vi "Coerce I64.vi"(4 "Rounding Mode (Round to Nearest))":T1, 8 "Value":i64, 9 "Increment":i64, 10 "Maximum":i64, 11 "Minimum":i64) -> (3 "Coerced Value":i64)   [LabVIEW 2020]
uses:
  Rounding Mode.ctl
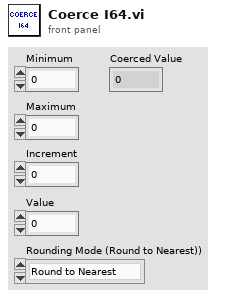
[diagram p1: front panel]
types:
  T1 = typedef "Rounding Mode.ctl" = enum16{"Round to Nearest", "Round to Lowest", "Round to Highest"}
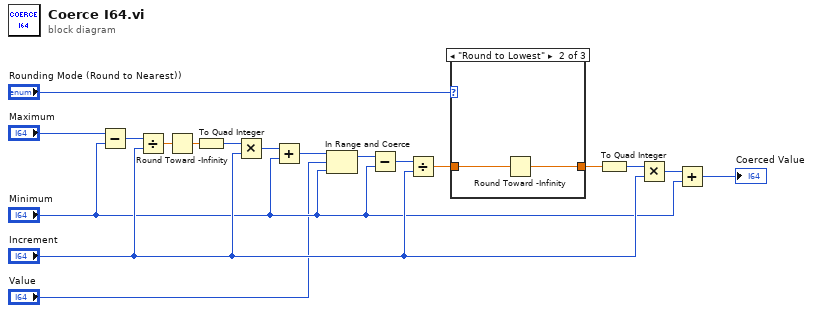
[diagram p0: block diagram]
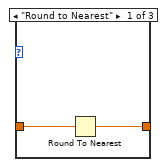
[diagram p2: hidden frame]
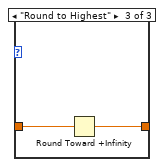
[diagram p3: hidden frame]
diagram:
  n1 = Subtract(x="Maximum", y="Minimum") -> (x-y=w14:i64)
  n2 = Divide(x=w14, y="Increment") -> (x/y=w13:dbl)
  n3 = Round Toward -Infinity(1:w13) -> (0:w8:dbl)
  n4 = To Quad Integer(1:w8) -> (0:w7:i64)
  n5 = Multiply(x=w7, y="Increment") -> (x*y=w6:i64)
  n6 = Add(x=w6, y="Minimum") -> (x+y=w10:i64)
  n7 = In Range and Coerce(upper limit=w10, x="Value", lower limit="Minimum") -> (coerced(x)=w16:i64)  [unwired: 1 out]
  n8 = Subtract(x=w16, y="Minimum") -> (x-y=w17:i64)
  n9 = Divide(x=w17, y="Increment") -> (x/y=w18:dbl)
  n10 = case shown="\"Round to Lowest\"" "Rounding Mode (Round to Nearest))" {
    tunnel: w18 -> [w20 w22 w24]
    tunnel: [w19 w21 w23] -> w4
    frame "Round to Nearest" {
      n11 = Round To Nearest(number=w20) -> (nearest integer value=w19:dbl)
    }
    frame "Round to Lowest" {
      n12 = Round Toward -Infinity(1:w22) -> (0:w21:dbl)
    }
    frame "Round to Highest" {
      n13 = Round Toward +Infinity(x=w24) -> (ceil(x): smallest int >= x=w23:dbl)
    }
  }
  n14 = To Quad Integer(1:w4) -> (0:w5:i64)
  n15 = Multiply(x=w5, y="Increment") -> (x*y=w3:i64)
  n16 = Add(x=w3, y="Minimum") -> (x+y=→"Coerced Value":i64)
